vi "Harmonic Spectrum.vi"(8 "error in (no error)":errorcluster, 9 "samples per cycle (192)":u16=192, 10 "maximum harmonic order (50)":u16=50, 11 "resampled data":T1[](array[typedef]) {"resampled signal" format="%.2f"; "times [s]" format="%.2f"}) -> (0 "error out":errorcluster, 3 "harmonic spectra":T2(array[cluster]))   [LabVIEW 2014, in "NI_EP_Power Measurement.lvlib"]
doc: "Calculates the fast Fourier transform (FFT) spectra from the resampled signals. This VI returns FFT spectra as complex spectra up to <B>maximum harmonic order</B>."
uses:
  <vilib>/addons/Electrical Power/Power Measurement/NI_EP_Power Measurement.lvlib
  <vilib>/addons/Electrical Power/Power Measurement/subVIs/ep_Resampled Data.ctl
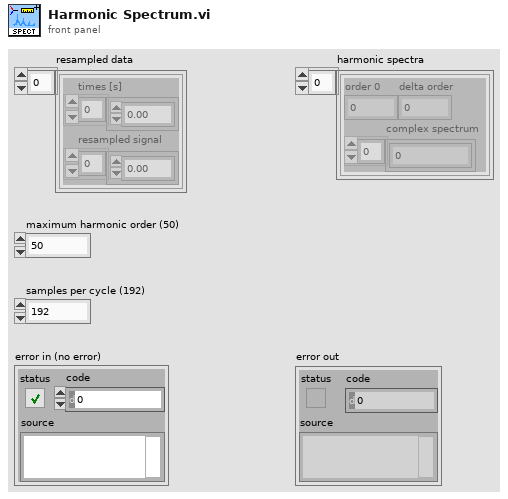
[diagram p1: front panel]
types:
  T1 = typedef "NI_EP_Power Measurement.lvlib/ep_Resampled Data.ctl" = cluster{"times [s]":dbl[], "resampled signal":dbl[]}
  T2 = cluster{"order 0":dbl, "delta order":dbl, "complex spectrum":cdb[]}[]
  T3 = cluster{"order 0":dbl, "delta order":dbl, "complex spectrum":cdb[]}
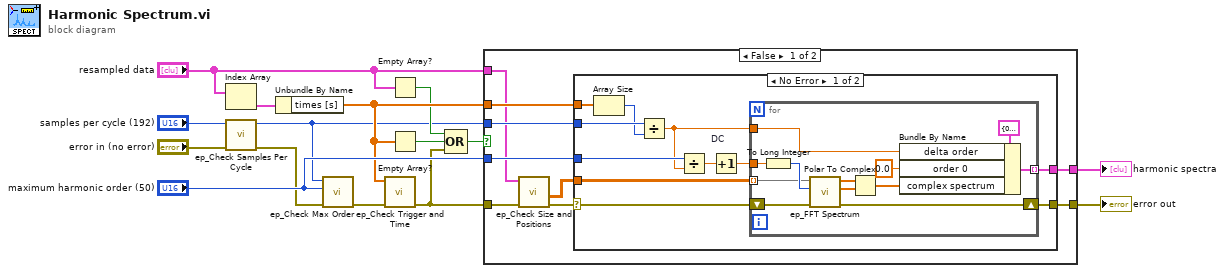
[diagram p0: block diagram]
diagram:
  n1 = Index Array(array="resampled data") -> (element=w11:T1)  [unwired: 1 in]
  n2 = call <vilib>:"ep_Check Samples Per Cycle.vi"("error in (no error)"="error in (no error)", "samples per cycle"="samples per cycle (192)") -> ("error out"=w4:errorcluster, "dup samples per cycle"=w1:u16)  [unwired: 8 in]
  n3 = Unbundle By Name(w11) -> ("times [s]"=w7:dbl[])
  n4 = call <vilib>:"ep_Check Max Order.vi"("error in (no error)"=w4, "maximum harmonic order"="maximum harmonic order (50)", "samples per cycle"=w1) -> ("error out"=w12:errorcluster)  [unwired: 8 in]
  n5 = call <vilib>:"ep_Check Trigger and Time.vi"("error in (no error)"=w12, "trigger/positions [s]"=w7) -> ("error out"=w9:errorcluster)  [unwired: 7 in, 2 out]
  n6 = Empty Array?(array="resampled data") -> (empty?=w5:bool)
  n7 = Empty Array?(array=w7) -> (empty?=w8:bool)
  n8 = Compound Arithmetic op=OR(w5, w8, w9) -> (w13:bool)
  n9 = case shown="False" w13 {
    tunnel: [w24 w49] -> w15
    tunnel: [w23 _] -> w14
    tunnel: "maximum harmonic order (50)" -> [w21 _]
    tunnel: w1 -> [w22 _]
    tunnel: w9 -> [w19 w49]
    tunnel: w7 -> [w18 _]
    tunnel: "resampled data" -> [w17 _]
    frame False {
      n10 = call <vilib>:"ep_Check Size and Positions.vi"("error in (no error)"=w19, "resampled data"=w17) -> ("error out"=w16:errorcluster, "resampled signal"=w20:dbl[][])  [unwired: 7 in, 1 out]
      n11 = case shown="No Error" w16 {
        selector: w16 -> [w28 w48]
        tunnel: [w35 w48] -> w24
        tunnel: [w34 _] -> w23
        tunnel: w22 -> [w27 _]
        tunnel: w21 -> [w33 _]
        tunnel: w20 -> [w32 _]
        tunnel: w18 -> [w29 _]
        frame No Error {
          n12 = Array Size(array=w29) -> (size(s)=w26:i32)
          n13 = Divide(x=w27, y=w26) -> (x/y=w25:dbl)
          n14 = Divide(x=w33, y=w25) -> (x/y=w31:dbl)
          n15 = Increment "DC"(x=w31) -> (x+1=w30:dbl)
          n16 = for {
            shift-right: [w44] -> w35
            shift-left: w28 -> [w45]
            tunnel: [w42] -> w34 mode=indexing
            tunnel: w30 -> [w47]
            tunnel: w25 -> [w38]
            tunnel: w32 -> [w36] mode=indexing
            n17 = To Long Integer(number=w47) -> (32bit integer=w46:i32)
            n18 = call <vilib>:"ep_FFT Spectrum.vi"("error in (no error)"=w45, "# of bins"=w46, "resampled signal"=w36) -> ("error out"=w44:errorcluster, "phase"=w40:dbl[], "magnitude"=w41:dbl[])  [unwired: 6 in]
            n19 = Polar To Complex(1:w40, 2:w41) -> (0:w39:cdb[])
            n20 = Bundle By Name(cluster=T3 {"order 0"=0.0, "delta order"=0.0, "complex spectrum"=[]} ("spectrum"), "delta order"=w38, "order 0"=0.0, "complex spectrum"=w39) -> (w42:T3)
          }
        }
        frame Error {
        }
      }
    }
    frame True {
    }
  }
  "error out" <- w15
  "harmonic spectra" <- w14
